vi "Add to Dictionary.vi"() -> ()   [LabVIEW 2015]
panel:
  out "Word":string
  in  "Add File":path=path "C:/Users/Ivan/Desktop/LabVIEW/Word_Game_LabVIEW_2015/Dictionary/russian_nouns.txt"
  out "Dictionary":string[](array[string])
  in  "Dictionary File":path=path "C:/Users/Ivan/Desktop/LabVIEW/Word_Game_LabVIEW_2015/Dictionary/Dictionary.txt"
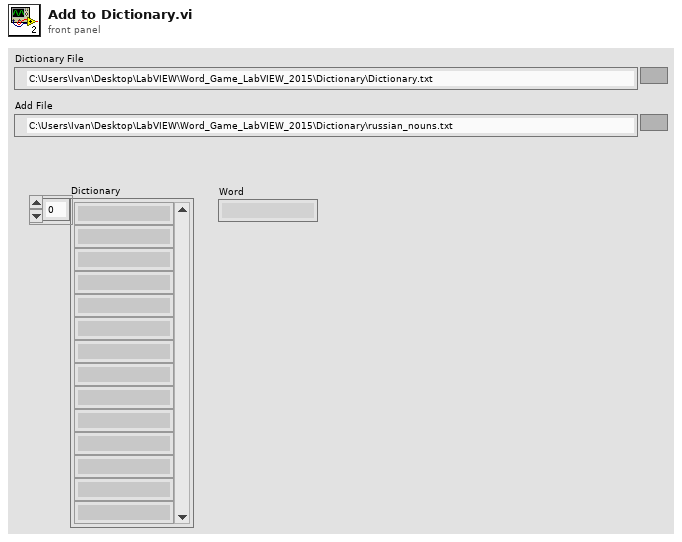
[diagram p1: front panel]
types:
  T1 = enum16{"open", "replace", "create", "open or create", "replace or create", "replace or create with confirmation"}
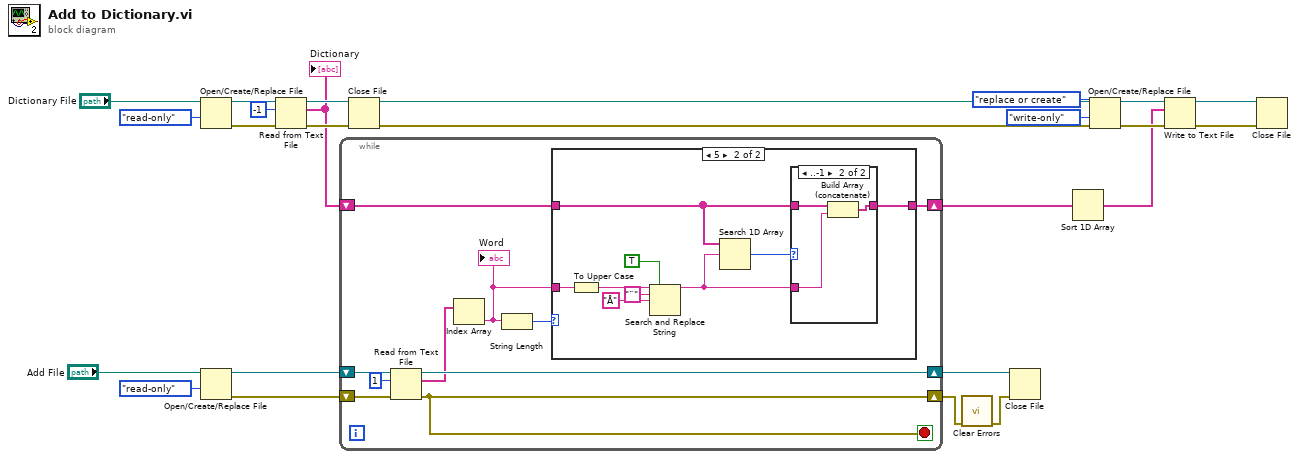
[diagram p0: block diagram]
diagram:
  n1 = Open/Create/Replace File(file path (use dialog)="Dictionary File", access (0:read/write)=enum16{"read/write", "read-only", "write-only"}."read-only") -> (refnum out=w23:refnum<file>, error out=w22:errorcluster)  [unwired: 4 in, 1 out]
  n2 = Open/Create/Replace File(file path (use dialog)="Add File", access (0:read/write)=enum16{"read/write", "read-only", "write-only"}."read-only") -> (refnum out=w6:refnum<file>, error out=w5:errorcluster)  [unwired: 4 in, 1 out]
  n3 = Read from Text File(file (use dialog)=w23, count=-1, error in=w22) -> (refnum out=w20:refnum<file>, text=w9:string[], error out=w19:errorcluster)  [unwired: 1 in, 1 out]
  "Dictionary" <- w9
  n4 = while {
    shift-right: [w34] -> w10
    shift-left: w9 -> [w35]
    shift-right: [w29] -> w4
    shift-left: w6 -> [w32]
    shift-right: [w30] -> w3
    shift-left: w5 -> [w31]
    stop <- w30 stop-if-true
    n5 = Read from Text File(file (use dialog)=w32, count=1, error in=w31) -> (refnum out=w29:refnum<file>, text=w28:string[], error out=w30:errorcluster)  [unwired: 1 in, 1 out]
    n6 = Index Array(array=w28) -> (element=w26:string)  [unwired: 1 in]
    "Word" <- w26
    n7 = String Length(string=w26) -> (length=w27:i32)
    n8 = case shown="5" w27 {
      tunnel: w35 -> [w36 w41]
      tunnel: [w36 w39] -> w34
      tunnel: w26 -> [_ w38]
      frame 0, Default {
      }
      frame 5 {
        n9 = To Upper Case(1:w38) -> (0:w37:string)
        n10 = Search and Replace String(replace all?=TRUE ("replace all? (F)"), input string=w37, search string="¨", replace string="Å" ("replace string (\"\")")) -> (result string=w40:string)  [unwired: 4 in, 3 out]
        n11 = Search 1D Array(1D array=w41, element=w40) -> (index of element=w42:i32)  [unwired: 1 in]
        n12 = case shown="..-1" w42 {
          tunnel: w41 -> [w46 w49]
          tunnel: w40 -> [_ w48]
          tunnel: [w46 w47] -> w39
          frame 0.. {
          }
          frame ..-1 {
            n13 = Build Array (concatenate)(w49, w48) -> (w47:string[])
          }
        }
      }
    }
  }
  n14 = Close File(refnum=w20, error in=w19) -> (path=w13:path, error out=w11:errorcluster)
  n15 = call <vilib>:"Clear Errors.vi"("error in (no error)"=w3) -> ("error out"=w2:errorcluster)  [unwired: 5 in, 1 out]
  n16 = Close File(refnum=w4, error in=w2) -> ()  [unwired: 2 out]
  n17 = Sort 1D Array(array=w10) -> (sorted array=w1:string[])
  n18 = Open/Create/Replace File(file path (use dialog)=w13, error in=w11, operation (0:open)=T1."replace or create", access (0:read/write)=enum16{"read/write", "read-only", "write-only"}."write-only") -> (refnum out=w15:refnum<file>, error out=w16:errorcluster)  [unwired: 2 in, 1 out]
  n19 = Write to Text File(file (use dialog)=w15, text=w1, error in=w16) -> (refnum out=w17:refnum<file>, error out=w18:errorcluster)  [unwired: 1 in, 1 out]
  n20 = Close File(refnum=w17, error in=w18) -> ()  [unwired: 2 out]
